vi "is_initialised.vi"(8 "error in (no error)":errorcluster, 11 "FPGAWrapperDL120115Galvo in":refnum<class "FPGAWrapperDL090211Galvo_grabber.lvclass">) -> (0 "error out":errorcluster, 2 "is initialised?":bool, 3 "FPGAWrapperDL120115Galvo out":refnum<class "FPGAWrapperDL090211Galvo_grabber.lvclass">)   [LabVIEW 2010, in "FPGAWrapperDL090211Galvo_grabber.lvclass"]
uses:
  FPGAWrapperDL090211Galvo_grabber.lvclass
  class_data.vi
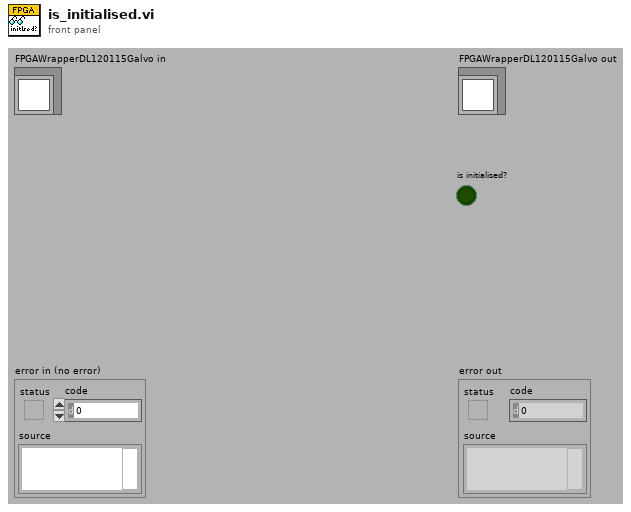
[diagram p1: front panel]
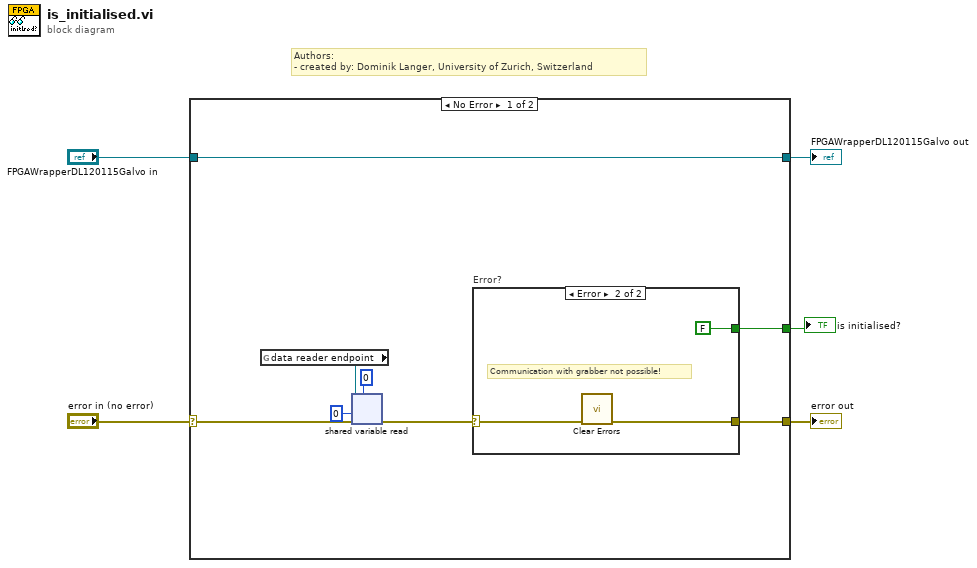
[diagram p0: block diagram]
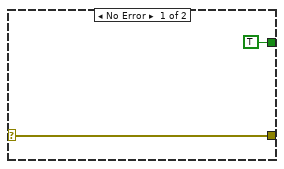
[diagram p2: hidden frame]
diagram:
  # "Authors: \n- created by: Dominik Langer, University of Zurich, Switzerland"
  n1 = case shown="No Error" "error in (no error)" {
    selector: "error in (no error)" -> [w9 w20]
    tunnel: [w6 w20] -> w4
    tunnel: [w13 w19] -> w2
    tunnel: "FPGAWrapperDL120115Galvo in" -> [w13 w19]
    tunnel: [w7 _] -> w1
    frame No Error {
      n2 = global read "class_data.vi" "data reader endpoint"() -> (w12:refnum<k21>)
      n3 = shared-variable-read(w12, w9, 0 ("timeout in ms (-1)"), 0 ("# elements (-1)")) -> (w8:errorcluster)  [unwired: 3 out]
      n4 = case "Error?" shown="Error" w8 {
        selector: w8 -> [w15 w17]
        tunnel: [TRUE FALSE] -> w7
        tunnel: [w15 w16] -> w6
        frame No Error {
        }
        frame Error {
          # "Communication with grabber not possible!"
          n5 = call <vilib>:"Clear Errors.vi"("error in (no error)"=w17) -> ("error out"=w16:errorcluster)  [unwired: 6 in]
        }
      }
    }
    frame Error {
    }
  }
  "error out" <- w4
  "FPGAWrapperDL120115Galvo out" <- w2
  "is initialised?" <- w1
